vi "Limit Switch Winch.vi"() -> ()   [LabVIEW 2013]
uses:
  <vilib>/Rock Robotics/WPI/Joystick/WPI_JoystickGetSetRefNum.vi
  Robot Global Data.vi
  Globals/Useful Values.vi
  Globals/Data for Dashboard.vi
  Globals/Homes.vi
  <vilib>/Utility/file.llb/Write To Spreadsheet File (DBL).vi
  <vilib>/addons/control/pid/pid.llb/PID (DBL).vi
  <vilib>/addons/control/pid/NI_PID_pid.lvlib
panel:
  out "Value":bool=TRUE
  in  "Pullback Speed":dbl=-1.0
  out "Motor Output":dbl
  out "Winch Voltage":dbl
  in  "PID gains":T1={"proportional gain (Kc)"=2.75, "integral time (Ti, min)"=0.0, "derivative time (Td, min)"=0.0} {"derivative time (Td, min)" format="%.3f"; "integral time (Ti, min)" format="%.3f"; "proportional gain (Kc)" format="%.3f"}
  # "PULLBACK SPEED NEEDS\nTO BE NEGATIVE OR ELSE"
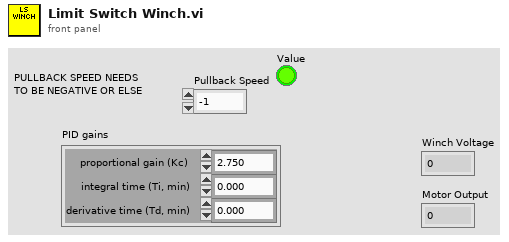
[diagram p1: front panel]
types:
  T1 = cluster{"proportional gain (Kc)":dbl, "integral time (Ti, min)":dbl, "derivative time (Td, min)":dbl}
  T2 = typedef "WPI_JoystickDevRef.ctl" = cluster{"Device":T3}
  T3 = typedef "WPI_JoystickDeviceEnum.ctl" = enum16{"USB 1", "USB 2", "USB 3", "USB 4", "Kinect 1", "Kinect 2"}
  T4 = typedef "WPI_MotorControlDeviceRef.ctl" = cluster{"DeviceStatus":errorcluster, "Type":enum16{"PWM", "CAN"}, "PWM":cluster{"Digital Module":T5, "PWM Channel":T6, "DeadBand":T7}, "CAN":cluster{"Device Number":u8, "Control Mode":T8, "Semaphore":T9, "Max Vout":dbl}, "Invert":bool, "TransformRef":T10, "InvTransformRef":T10}
  T5 = typedef "FPGA_TypedefDigitalModule.ctl" = enum16{"Digital Module 1", "Digital Module 2"}
  T6 = typedef "FPGA_DIOPWMChannel.ctl" = enum8{"PWM 1", "PWM 2", "PWM 3", "PWM 4", "PWM 5", "PWM 6", "PWM 7", "PWM 8", "PWM 9", "PWM 10", "Invalid"}
  T7 = typedef "WPI_PWMDeadband.ctl" = cluster{"Name":string, "maxPositivePwm":i32, "minPositivePwm":i32, "centerPwm":i32, "maxNegativePwm":i32, "minNegativePwm":i32, "angularRange":u16}
  T8 = typedef "WPI_CANJaguar_ControlMode.ctl" = enum8{"Percent VBus", "Current", "Speed", "Position", "Voltage"}
  T9 = typedef "Semaphore RefNum" = refnum<k1>
  T10 = typedef "WPI_PWMTransform_ConPane.ctl" = refnum<vi>
  T11 = typedef "WPI_DigitalInputDevRef.ctl" = cluster{"DevStatus":errorcluster, "DIO Channel":T12, "Digital Module":T5}
  T12 = typedef "FPGA_DIOChannel.ctl" = enum8{"DIO 1", "DIO 2", "DIO 3", "DIO 4", "DIO 5", "DIO 6", "DIO 7", "DIO 8", "DIO 9", "DIO 10", "DIO 11", "DIO 12", "DIO 13", "DIO 14", "Invalid"}
  T13 = typedef "WPI_AnalogChannelDevRef.ctl" = cluster{"DevStatus":errorcluster, "Analog Module":T14, "Analog Channel":T15}
  T14 = typedef "FPGA_TypedefAnalogModule.ctl" = enum16{"Analog Module 1", "Analog Module 2"}
  T15 = typedef "FPGA_AIChannel.ctl" = enum8{"AI 1", "AI 2", "AI 3", "AI 4", "AI 5", "AI 6", "AI 7", "AI 8", "Invalid"}
  T16 = typedef "WPI_DriverStationRobotMode2.ctl" = enum16{"Autonomous Disabled", "Autonomous Enabled", "Teleop Disabled", "Teleop Enabled", "Timeout", "Finish", "Test Disabled", "Test Enabled"}
  T17 = typedef "WPI_JoystickButtonState.ctl" = cluster{"Button 1":bool, "Button 2":bool, "Button 3":bool, "Button 4":bool, "Button 5":bool, "Button 6":bool, "Button 7":bool, "Button 8":bool, "Button 9":bool, "Button 10":bool, "Button 11":bool, "Button 12":bool}
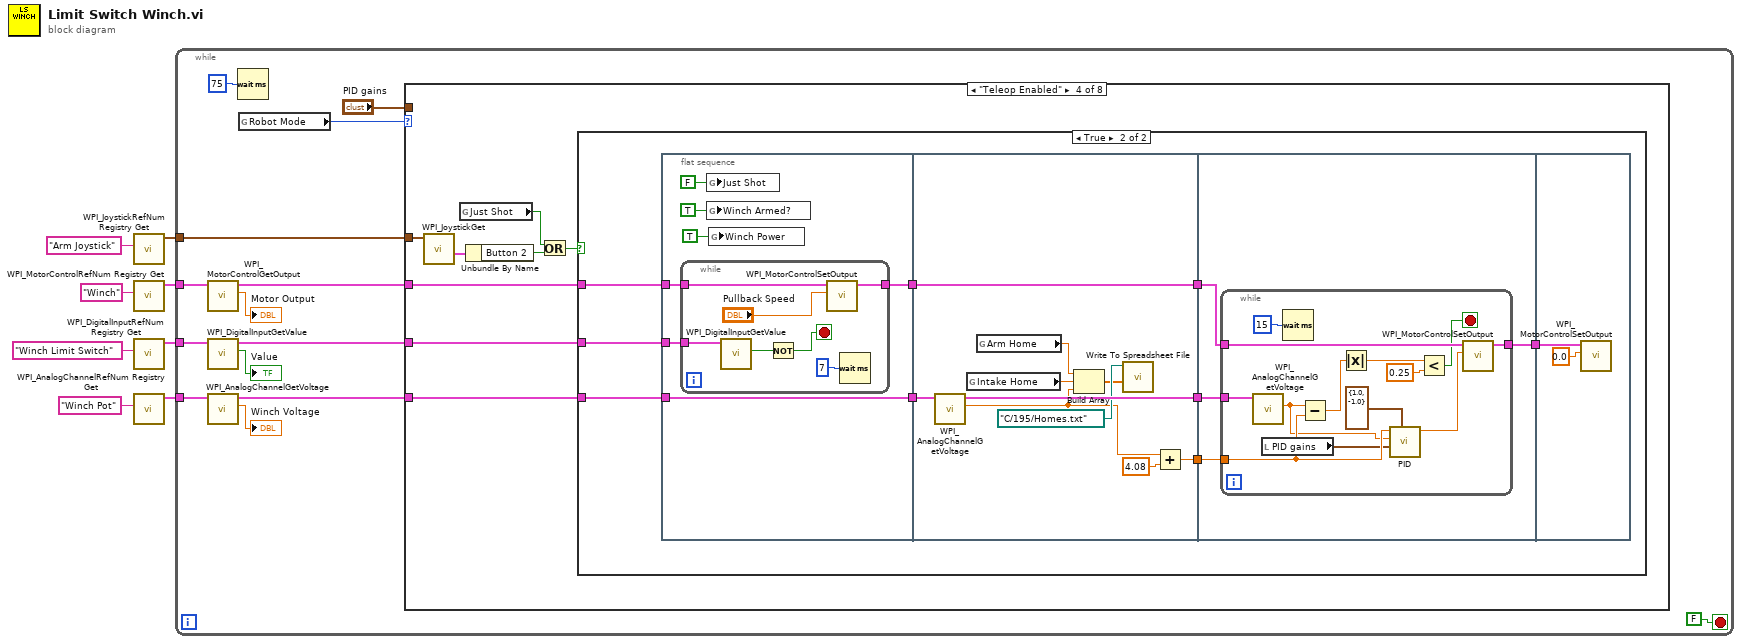
[diagram p0: block diagram]
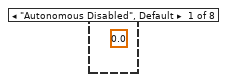
[diagram p2: hidden frame]
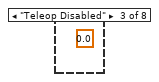
[diagram p4: hidden frame]
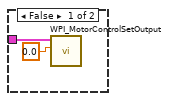
[diagram p5: hidden frame]
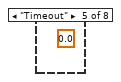
[diagram p6: hidden frame]
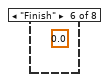
[diagram p7: hidden frame]
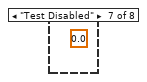
[diagram p8: hidden frame]
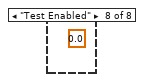
[diagram p9: hidden frame]
diagram:
  n1 = call <vilib>:"WPI_JoystickRefNum Registry Get.vi"("refnum name"="Arm Joystick") -> ("JoystickDevRef"=w3:T2)  [unwired: 9 in, 1 out]
  n2 = call <vilib>:"WPI_MotorControlRefNum Registry Get.vi"("refnum name"="Winch") -> ("MotorControlDevRef"=w5:T4)  [unwired: 9 in, 1 out]
  n3 = call <vilib>:"WPI_DigitalInputRefNum Registry Get.vi"("refnum name"="Winch Limit Switch") -> ("DigitalInputDevRef"=w2:T11)  [unwired: 9 in, 1 out]
  n4 = call <vilib>:"WPI_AnalogChannelRefNum Registry Get.vi"("refnum name"="Winch Pot") -> ("AIDeviceRef"=w8:T13)  [unwired: 9 in, 1 out]
  n5 = while {
    tunnel: w8 -> [w20]
    tunnel: w5 -> [w14]
    tunnel: w3 -> [w16]
    tunnel: w2 -> [w11]
    stop <- FALSE stop-if-true
    n6 = call <vilib>:"WPI_MotorControlGetOutput.vi"("MotorControlDevRef"=w14) -> ("Output"=→"Motor Output":dbl, "MotorControlDevRef"=w12:T4)  [unwired: 8 in, 1 out]
    n7 = call <vilib>:"WPI_DigitalInputGetValue.vi"("DigitalInputDevRef"=w11) -> ("Value"=→"Value":bool, "DigitalInputDevRef"=w10:T11)  [unwired: 8 in, 1 out]
    n8 = call <vilib>:"WPI_AnalogChannelGetVoltage.vi"("AIDeviceRef"=w20) -> ("Voltage"=→"Winch Voltage":dbl, "AIDeviceRef"=w15:T13)  [unwired: 8 in, 1 out]
    n9 = Wait (ms)(milliseconds to wait=u32 75) -> ()  [unwired: 1 out]
    n10 = global read "Robot Global Data.vi" "Robot Mode"() -> (w19:T16)
    n11 = case shown="\"Teleop Enabled\"" w19 {
      tunnel: w12 -> [_ _ _ w27 _ _ _ _]
      tunnel: "PID gains" -> [_ _ _ _ _ _ _ _]
      tunnel: w16 -> [_ _ _ w30 _ _ _ _]
      tunnel: w10 -> [_ _ _ w28 _ _ _ _]
      tunnel: w15 -> [_ _ _ w26 _ _ _ _]
      frame "Autonomous Disabled", Default {
        (unwired) 0.0 ("Motor Output")
      }
      frame "Autonomous Enabled" {
      }
      frame "Teleop Disabled" {
        (unwired) 0.0 ("Motor Output")
      }
      frame "Teleop Enabled" {
        n12 = call <vilib>:"WPI_JoystickGet.vi"("JoystickDevRef"=w30) -> ("Buttons"=w29:T17)  [unwired: 4 in, 2 out]
        n13 = global read "Useful Values.vi" "Just Shot"() -> (w24:bool)
        n14 = Unbundle By Name(w29) -> ("Button 2"=w25:bool)
        n15 = Or(x=w24, y=w25) -> (x .or. y?=w23:bool)
        n16 = case shown="True" w23 {
          tunnel: w28 -> [_ w41]
          tunnel: w27 -> [w31 w40]
          tunnel: w26 -> [_ w34]
          frame False {
            n17 = call <vilib>:"WPI_MotorControlSetOutput.vi"("Output"=0.0, "MotorControlDevRef"=w31) -> ()  [unwired: 7 in, 3 out]
          }
          frame True {
            n18 = flat-sequence {
              tunnel: w41 -> [w48]
              tunnel: w40 -> [w47]
              tunnel: [w46] -> w39
              tunnel: [w45] -> w35
              tunnel: w34 -> [w45]
              tunnel: w39 -> [w65]
              tunnel: [w65] -> w38
              tunnel: [w64] -> w37
              tunnel: w35 -> [w63]
              tunnel: [w62] -> w33
              tunnel: w38 -> [w69]
              tunnel: w37 -> [w67]
              tunnel: [w66] -> w36
              tunnel: w33 -> [w68]
              tunnel: w36 -> [w84]
              frame #0 {
                n19 = while {
                  tunnel: w48 -> [w55]
                  tunnel: w47 -> [w51]
                  tunnel: [w50] -> w46
                  stop <- w49 stop-if-true
                  n20 = call <vilib>:"WPI_DigitalInputGetValue.vi"("DigitalInputDevRef"=w55) -> ("Value"=w54:bool)  [unwired: 8 in, 2 out]
                  n21 = Not(x=w54) -> (.not. x?=w49:bool)
                  n22 = call <vilib>:"WPI_MotorControlSetOutput.vi"("Output"="Pullback Speed", "MotorControlDevRef"=w51) -> ("MotorControlDevRef"=w50:T4)  [unwired: 7 in, 2 out]
                  n23 = Wait (ms)(milliseconds to wait=u32 7) -> ()  [unwired: 1 out]
                }
                n24 = global write "Useful Values.vi" "Just Shot"(FALSE ("Just Shot")) -> ()
                n25 = global write "Data for Dashboard.vi" "Winch Armed?"(TRUE ("Loaded")) -> ()
                n26 = global write "Data for Dashboard.vi" "Winch Power"(TRUE ("Loaded")) -> ()
              }
              frame #1 {
                n27 = call <vilib>:"WPI_AnalogChannelGetVoltage.vi"("AIDeviceRef"=w63) -> ("Voltage"=w56:dbl, "AIDeviceRef"=w64:T13)  [unwired: 8 in, 1 out]
                n28 = global read "Homes.vi" "Intake Home"() -> (w57:dbl)
                n29 = global read "Homes.vi" "Arm Home"() -> (w59:dbl)
                n30 = Build Array(w59, w57, w56) -> (w58:dbl[])
                n31 = call-poly <vilib>:"Write To Spreadsheet File.vi"("1D data"=w58, "file path (dialog if empty)"=path "C:/195/Homes.txt") -> ()  [unwired: 6 in, 1 out]
                n32 = Add(x=w56, y=4.08) -> (x+y=w62:dbl)
              }
              frame #2 {
                n33 = while {
                  tunnel: w69 -> [w82]
                  tunnel: w68 -> [w75]
                  tunnel: w67 -> [w77]
                  tunnel: [w73] -> w66
                  stop <- w79 stop-if-true
                  n34 = call <vilib>:"WPI_AnalogChannelGetVoltage.vi"("AIDeviceRef"=w77) -> ("Voltage"=w74:dbl)  [unwired: 8 in, 2 out]
                  n35 = local read "PID gains"() -> (w72:T1)
                  n36 = Wait (ms)(milliseconds to wait=u32 15) -> ()  [unwired: 1 out]
                  n37 = Subtract(x=w74, y=w75) -> (x-y=w81:dbl)
                  n38 = Absolute Value(x=w81) -> (abs(x)=w80:dbl)
                  n39 = call-poly <vilib>:"PID.vi"("output range"=cluster{"output high":dbl, "output low":dbl} {"output high"=1.0, "output low"=-1.0}, "PID gains"=w72, "process variable"=w74, "setpoint"=w75) -> ("output"=w70:dbl)  [unwired: 6 in, 1 out]
                  n40 = Less?(x=w80, y=0.25) -> (x < y?=w79:bool)
                  n41 = call <vilib>:"WPI_MotorControlSetOutput.vi"("Output"=w70, "MotorControlDevRef"=w82) -> ("MotorControlDevRef"=w73:T4)  [unwired: 7 in, 2 out]
                }
              }
              frame #3 {
                n42 = call <vilib>:"WPI_MotorControlSetOutput.vi"("Output"=0.0, "MotorControlDevRef"=w84) -> ()  [unwired: 7 in, 3 out]
              }
            }
          }
        }
      }
      frame "Timeout" {
        (unwired) 0.0 ("Motor Output")
      }
      frame "Finish" {
        (unwired) 0.0 ("Motor Output")
      }
      frame "Test Disabled" {
        (unwired) 0.0 ("Motor Output")
      }
      frame "Test Enabled" {
        (unwired) 0.0 ("Motor Output")
      }
    }
  }
